vi "Test#CMDExecute.vi"(3 "ProgramRef":refnum<vi>, 4 "Command":string[](array[string]), 5 "ThreadsQueue":refnum<queue>[](array[refnum]), 6 "ThreadNo.":u32, 7 "ThreadModReceive":refnum<queue>[](array[refnum]), 8 "StackIn":cluster{"Program":i32, "Prog Index":i32}[](array[cluster]), 9 "ThreadInfoIn":T1) -> (0 "StackOut":cluster{"Program":i32, "Prog Index":i32}[](array[cluster]), 1 "ThreadInfoOut":T1, 2 "ErrorCode":string)   [LabVIEW 2020]
uses:
  MainFrame/Global.vi
panel:
  out "KeyFind?":bool[](array[boolean])
  out "KeyValues":string[](array[string])
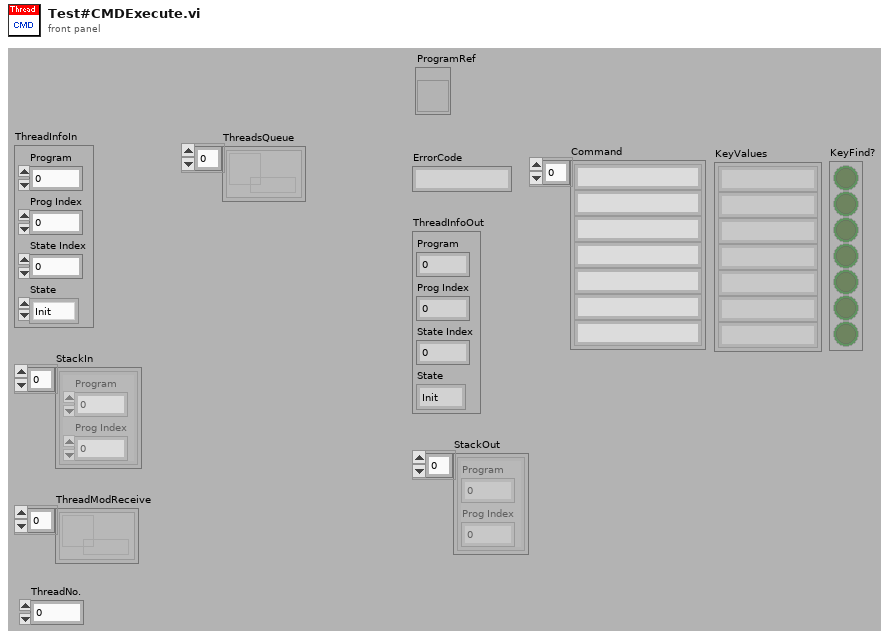
[diagram p1: front panel]
types:
  T1 = cluster{"Program":i32, "Prog Index":i32, "State Index":i32, "State":enum16{"Init", "Idle", "Auto Start", "Auto Running", "Step Start", "Step Running", "Suspend", "Restart", "Stop", "Reset"}}
  T2 = cluster{"指令":string, "代碼":string, "參數長度":i32, "乘數":dbl, "加數":dbl}[]
  T3 = cluster{"Command":string, "Parameter":string, "queue out":refnum<queue>}
  T4 = cluster{"指令":string, "代碼":string, "參數長度":i32, "乘數":dbl, "加數":dbl}[][]
  T5 = cluster{"指令":string, "代碼":string, "參數長度":i32, "乘數":dbl, "加數":dbl}
  T6 = enum16{"Init", "Idle", "Auto Start", "Auto Running", "Step Start", "Step Running", "Suspend", "Restart", "Stop", "Reset"}
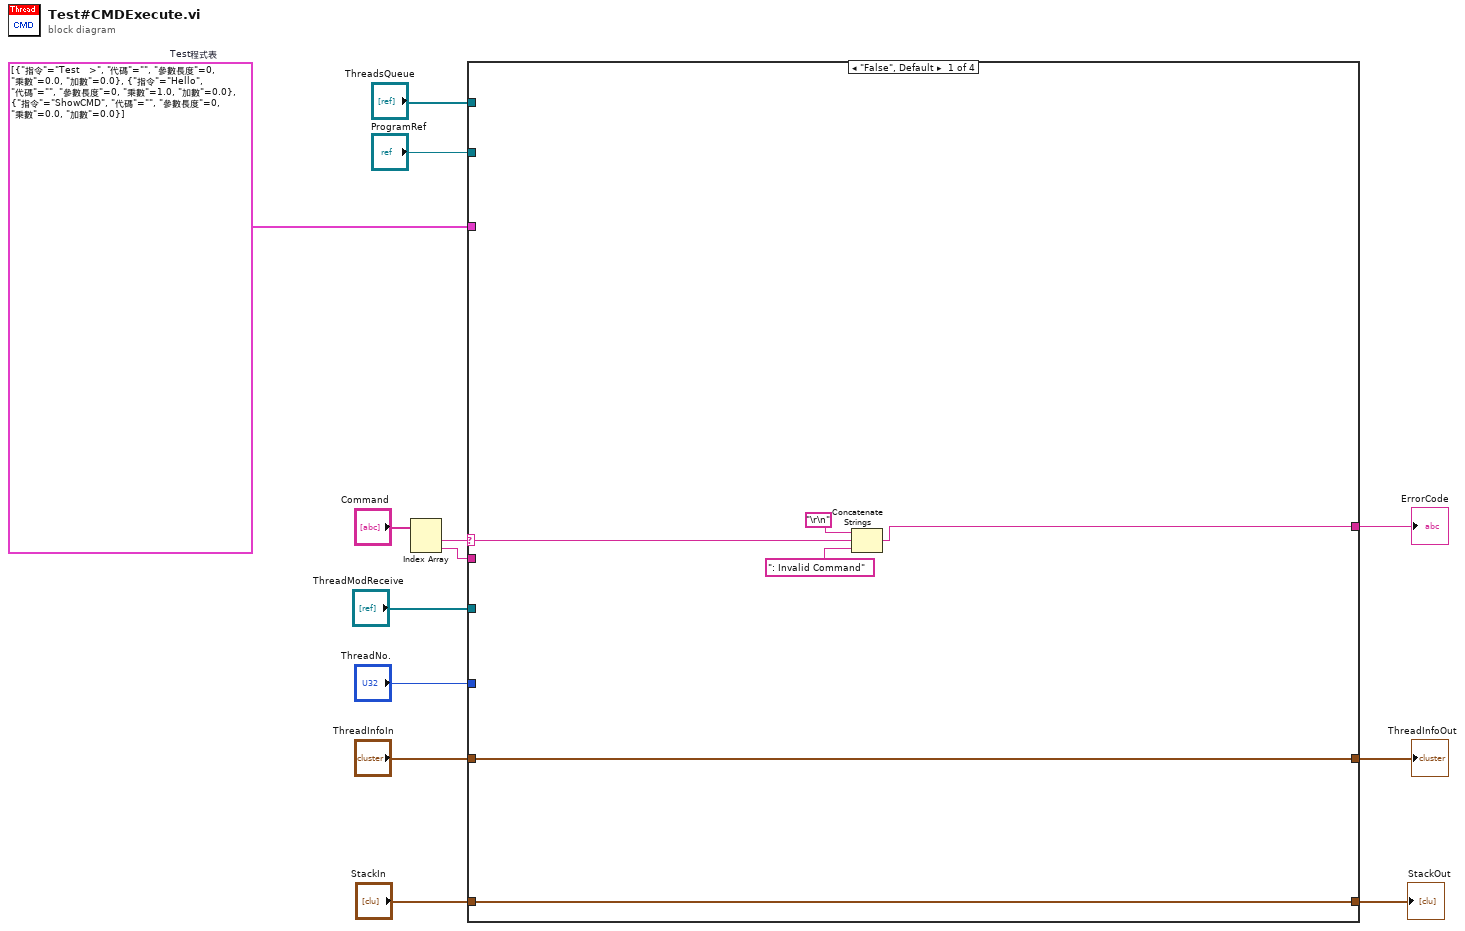
[diagram p0: block diagram]
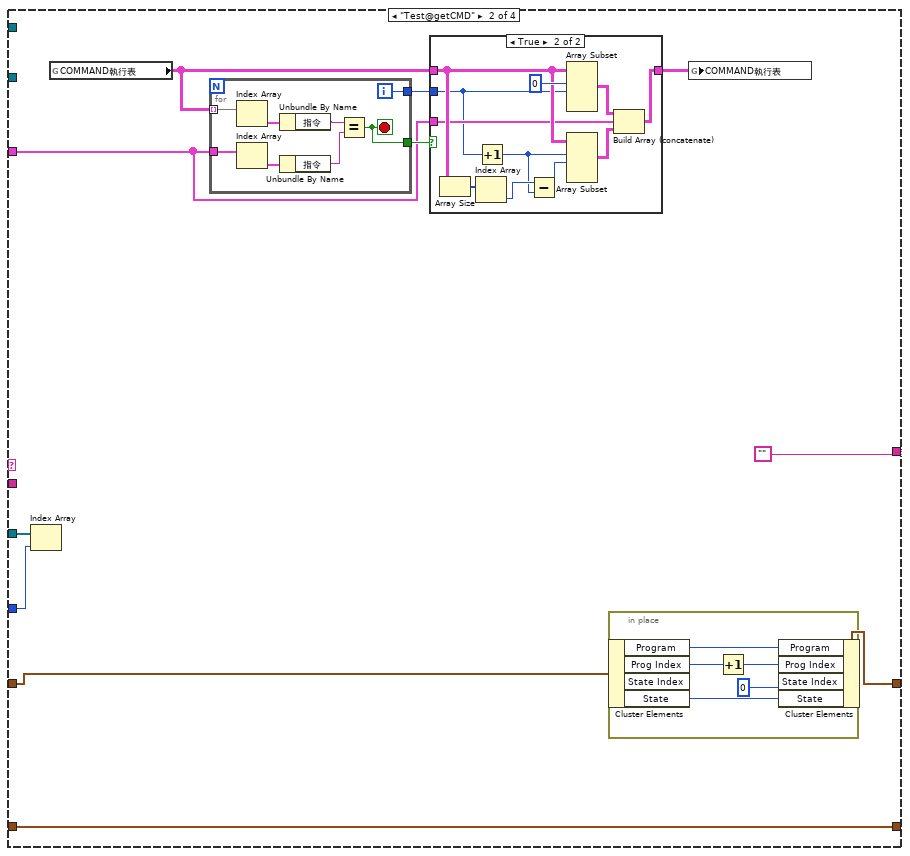
[diagram p2: hidden frame]
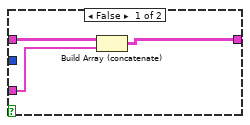
[diagram p3: hidden frame]
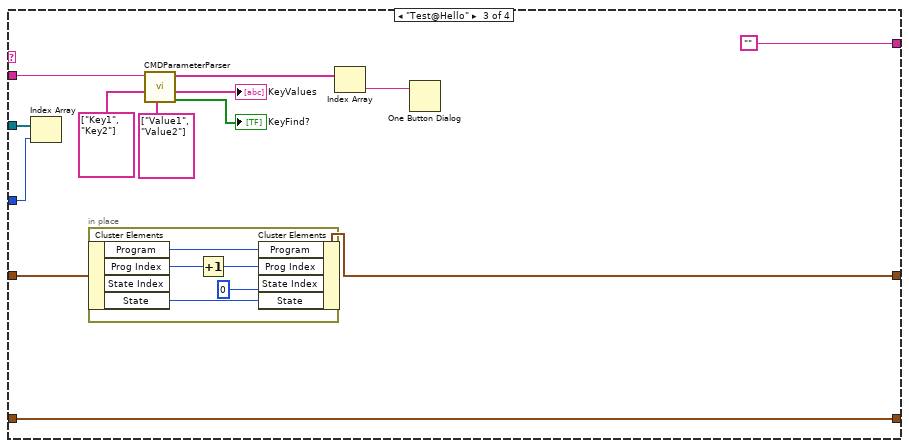
[diagram p4: hidden frame]
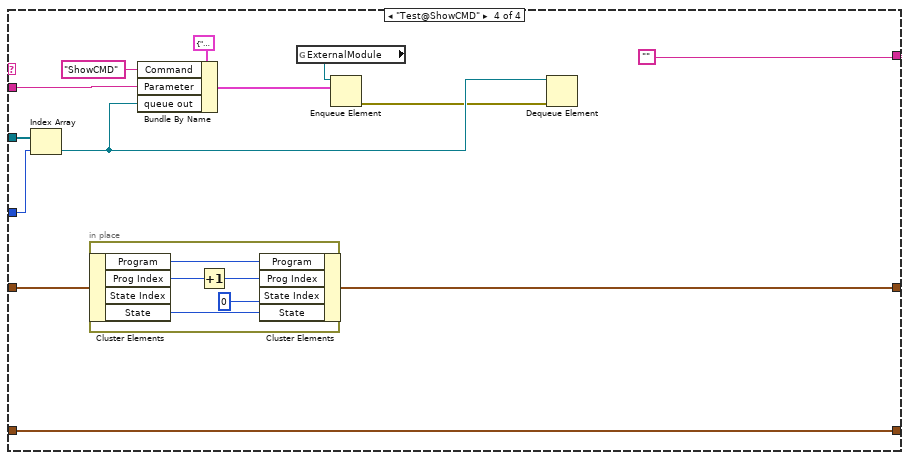
[diagram p5: hidden frame]
diagram:
  w2 = T2 [{"指令"="Test   >", "代碼"="", "參數長度"=0, "乘數"=0.0, "加數"=0.0}, {"指令"="Hello", "代碼"="", "參數長度"=0, "乘數"=1.0, "加數"=0.0}, {"指令"="ShowCMD", "代碼"="", "參數長度"=0, "乘數"=0.0, "加數"=0.0}]  # Test程式表
  n1 = Index Array(array="Command") -> (element #1=w10:string, element #2=w8:string)  [unwired: 2 in]
  n2 = case shown="\"False\", Default" w10 {
    selector: w10 -> [w17 _ _ _]
    tunnel: "ThreadModReceive" -> [_ w30 w70 w88]
    tunnel: [w19 w28 w68 w86] -> w5
    tunnel: "ThreadInfoIn" -> [w19 w27 w67 w85]
    tunnel: "ThreadNo." -> [_ w29 w69 w87]
    tunnel: w8 -> [_ _ w64 w82]
    tunnel: "ThreadsQueue" -> [_ _ _ _]
    tunnel: [w14 "" "" ""] -> w11
    tunnel: [w18 w26 w66 w84] -> w12
    tunnel: "StackIn" -> [w18 w26 w66 w84]
    tunnel: w2 -> [_ w22 _ _]
    tunnel: "ProgramRef" -> [_ _ _ _]
    frame "False", Default {
      n3 = Concatenate Strings("\r\n", w17, ": Invalid Command" ("string")) -> (w14:string)
    }
    frame "Test@getCMD" {
      n4 = Index Array(array=w30, index=w29) -> ()  [unwired: 1 out]
      n5 = global read "Global.vi" "COMMAND執行表"() -> (w21:T4)
      n6 = for {
        tunnel: w21 -> [w50] mode=indexing
        tunnel: w22 -> [w51]
        tunnel: [w46] -> w23
        tunnel: [w45] -> w24
        i -> [w46]
        stop <- w45 stop-if-true
        n7 = Index Array(array=w50) -> (element=w52:T5)  [unwired: 1 in]
        n8 = Index Array(array=w51) -> (element=w49:T5)  [unwired: 1 in]
        n9 = Unbundle By Name(w52) -> ("指令"=w48:string)
        n10 = Unbundle By Name(w49) -> ("指令"=w47:string)
        n11 = Equal?(x=w48, y=w47) -> (x = y?=w45:bool)
      }
      n12 = case shown="True" w24 {
        tunnel: w23 -> [_ w35]
        tunnel: w22 -> [w32 w38]
        tunnel: w21 -> [w33 w43]
        tunnel: [w31 w36] -> w20
        frame False {
          n13 = Build Array (concatenate)(w33, w32) -> (w31:T4)
        }
        frame True {
          n14 = Array Size(array=w43) -> (size(s)=w42:i32[])
          n15 = Index Array(array=w42) -> (element=w41:i32)  [unwired: 1 in]
          n16 = Increment(x=w35) -> (x+1=w34:i32)
          n17 = Subtract(x=w41, y=w34) -> (x-y=w40:i32)
          n18 = Array Subset(array=w43, index (row)=0 ("index"), length (row)=w35) -> (w39:T4)  [unwired: 2 in]
          n19 = Array Subset(array=w43, index (row)=w34, length (row)=w40) -> (w37:T4)  [unwired: 2 in]
          n20 = Build Array (concatenate)(w39, w38, w37) -> (w36:T4)
        }
      }
      n21 = in-place {
        n22 = in-place-cluster #1(w27) -> ("Program"=w57:i32, "Prog Index"=w55:i32, "State"=w53:T6)  [unwired: 1 out]
        n23 = Increment(x=w55) -> (x+1=w56:i32)
        n24 = in-place-cluster #1("Program"=w57, "Prog Index"=w56, "State Index"=0, "State"=w53) -> (w28:T1)
      }
      n25 = global write "Global.vi" "COMMAND執行表"(w20) -> ()
    }
    frame "Test@Hello" {
      n26 = Index Array(array=w70, index=w69) -> ()  [unwired: 1 out]
      n27 = in-place {
        n28 = in-place-cluster #2(w67) -> ("Program"=w75:i32, "Prog Index"=w73:i32, "State"=w71:T6)  [unwired: 1 out]
        n29 = Increment(x=w73) -> (x+1=w74:i32)
        n30 = in-place-cluster #2("Program"=w75, "Prog Index"=w74, "State Index"=0, "State"=w71) -> (w68:T1)
      }
      n31 = call "CMDParameterParser.vi"("DeafultValues"=string[] ["Value1", "Value2"] ("RequiredKeys"), "RequiredKeys"=string[] ["Key1", "Key2"], "CMDParameter"=w64) -> ("KeyFind?"=→"KeyFind?":bool[], "KeyValues"=→"KeyValues":string[], "Input"=w63:string[])  [unwired: 6 in]
      n32 = Index Array(array=w63) -> (element=w58:string)  [unwired: 1 in]
      n33 = One Button Dialog(message=w58) -> ()  [unwired: 1 in, 1 out]
    }
    frame "Test@ShowCMD" {
      n34 = Index Array(array=w88, index=w87) -> (element=w81:refnum<queue>)
      n35 = in-place {
        n36 = in-place-cluster #3(w85) -> ("Program"=w93:i32, "Prog Index"=w91:i32, "State"=w89:T6)  [unwired: 1 out]
        n37 = Increment(x=w91) -> (x+1=w92:i32)
        n38 = in-place-cluster #3("Program"=w93, "Prog Index"=w92, "State Index"=0, "State"=w89) -> (w86:T1)
      }
      n39 = Bundle By Name(cluster=T3 {"Command"="", "Parameter"="", "queue out"=refnum} ("CMD"), "Command"="ShowCMD", "Parameter"=w82, "queue out"=w81) -> (w78:T3)
      n40 = global read "Global.vi" "ExternalModule"() -> (w80:refnum<queue>)
      n41 = Enqueue Element(queue=w80, element=w78) -> (error out=w76:errorcluster)  [unwired: 2 in, 2 out]
      n42 = Dequeue Element(queue=w81, error in (no error)=w76) -> ()  [unwired: 1 in, 4 out]
    }
  }
  "StackOut" <- w12
  "ErrorCode" <- w11
  "ThreadInfoOut" <- w5
